vi "Determine Sector Edge Location.vi"(11 "Preanalysis Stage":bool) -> (2 "Left Sector Edge":u8, 3 "Right Sector Edge":u8)   [LabVIEW 2013]
doc: "Takes the average sector intensities and compares each average to the threshold value to determine which sector the edge is located in."
uses:
  Globals/Accumulated Sector Intensity.vi
  Globals/Sector Parameter Global.vi
  <vilib>/rvi/FIFO/Fifo_Resource/nirvififoEmulationReadFpgaImpl.vi
  <vilib>/rvi/DataTransferAndStorage/Container/Common/niFpgaContainerGetUniqueNameForEmu.vi
  <vilib>/rvi/interface/RandomDataEmulation/nirviRandomDataFPGAFIFO.vi
  <vilib>/rvi/interface/RandomDataEmulation/niFpgaRandomDataHandleErrors.vi
  <vilib>/rvi/DataTransferAndStorage/Container/XNode/niFpgaContainer.xnode
  <vilib>/rvi/FIFO/Fifo_Resource/nirvififoEmulationRead.vi
  <vilib>/rvi/interface/RandomDataEmulation/nirviRandomDataFpgaReadWriteTemplate.vi
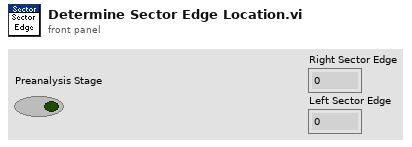
[diagram p1: front panel]
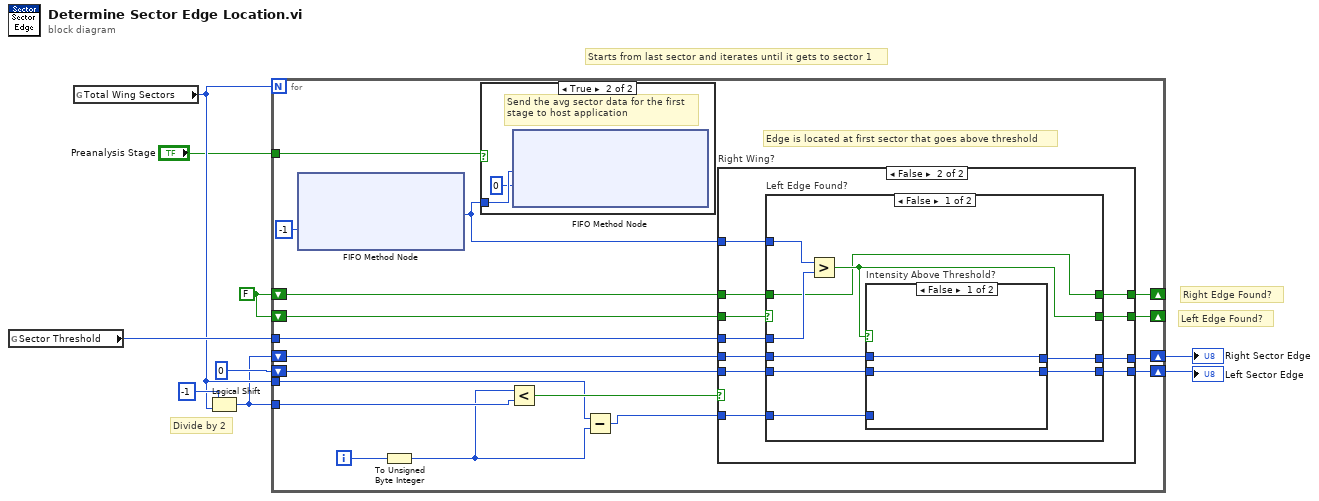
[diagram p0: block diagram]
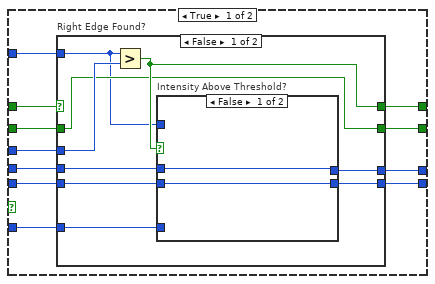
[diagram p3: hidden frame]
diagram:
  w6 = FALSE ("Left Edge Found?")
  # "Starts from last sector and iterates until it gets to sector 1"
  # "Left Edge Found?"
  # "Right Edge Found?"
  # "Divide by 2"
  n1 = global read "Sector Parameter Global.vi" "Sector Threshold"() -> (w4:u8)
  n2 = global read "Accumulated Sector Intensity.vi" "Total Wing Sectors"() -> (w3:u8)
  n3 = Logical Shift(y=i16 -1, x=w3) -> (x << y=w1:u8)
  n4 = for {
    N: w3 -> [_]
    tunnel: w4 -> [w25]
    tunnel: w1 -> [w26]
    shift-right: [w23] -> _
    shift-left: w6 -> [w24]
    shift-right: [w16] -> _
    shift-left: w6 -> [w17]
    shift-right: [w21] -> w9
    shift-left: w1 -> [w20]
    shift-right: [w19] -> w8
    shift-left: u8 0 ("Total Wing Sectors") -> [w18]
    tunnel: w3 -> [w13]
    tunnel: "Preanalysis Stage" -> [w10]
    i -> [w22]
    # "Edge is located at first sector that goes above threshold"
    n5 = xnode ("FIFO Method Node")("Timeout"=-1) -> ("Element"=w15:u8)  [unwired: 1 in, 2 out]
    n6 = To Unsigned Byte Integer(number=w22) -> (unsigned 8bit integer=w12:u8)
    n7 = case shown="True" w10 {
      tunnel: w15 -> [_ w29]
      frame False {
      }
      frame True {
        # "Send the avg sector data for the first\nstage to host application"
        n8 = xnode ("FIFO Method Node")("Element"=w29, "Timeout"=0) -> ()  [unwired: 1 in, 2 out]
      }
    }
    n9 = Less?(x=w12, y=w26) -> (x < y?=w27:bool)
    n10 = Subtract(x=w13, y=w12) -> (x-y=w11:u8)
    n11 = case "Right Wing?" shown="False" w27 {
      tunnel: w15 -> [w39 w68]
      tunnel: w25 -> [w38 w67]
      tunnel: w24 -> [w40 w59]
      tunnel: [w37 w66] -> w23
      tunnel: w11 -> [w36 w65]
      tunnel: [w35 w64] -> w21
      tunnel: w20 -> [w34 w63]
      tunnel: [w33 w62] -> w19
      tunnel: w18 -> [w32 w61]
      tunnel: w17 -> [w31 w60]
      tunnel: [w30 w58] -> w16
      frame True {
        n12 = case "Right Edge Found?" shown="False" w40 {
          selector: w40 -> [_ w54]
          tunnel: w39 -> [w41 _]
          tunnel: w38 -> [w49 _]
          tunnel: [w48 w54] -> w37
          tunnel: w36 -> [w47 _]
          tunnel: [w46 w57] -> w35
          tunnel: w34 -> [w45 w57]
          tunnel: [w44 w56] -> w33
          tunnel: w32 -> [w43 w56]
          tunnel: w31 -> [w42 w55]
          tunnel: [w42 w55] -> w30
          frame False {
            n13 = Greater?(x=w41, y=w49) -> (0:w48:bool)
            n14 = case "Intensity Above Threshold?" shown="False" w48 {
              tunnel: w47 -> [_ w52]
              tunnel: [w51 w52] -> w46
              tunnel: w45 -> [w51 _]
              tunnel: [w50 w53] -> w44
              tunnel: w43 -> [w50 w53]
              tunnel: w41 -> [_ _]
              frame False {
              }
              frame True {
              }
            }
          }
          frame True {
          }
        }
      }
      frame False {
        n15 = case "Left Edge Found?" shown="False" w60 {
          selector: w60 -> [_ w82]
          tunnel: w68 -> [w69 _]
          tunnel: w67 -> [w77 _]
          tunnel: [w70 w83] -> w66
          tunnel: w65 -> [w76 _]
          tunnel: [w75 w85] -> w64
          tunnel: w63 -> [w74 w85]
          tunnel: [w73 w84] -> w62
          tunnel: w61 -> [w72 w84]
          tunnel: w59 -> [w70 w83]
          tunnel: [w71 w82] -> w58
          frame False {
            n16 = Greater?(x=w69, y=w77) -> (0:w71:bool)
            n17 = case "Intensity Above Threshold?" shown="False" w71 {
              tunnel: w76 -> [_ w80]
              tunnel: [w79 w81] -> w75
              tunnel: w74 -> [w79 w81]
              tunnel: [w78 w80] -> w73
              tunnel: w72 -> [w78 _]
              frame False {
              }
              frame True {
              }
            }
          }
          frame True {
          }
        }
      }
    }
  }
  "Right Sector Edge" <- w9
  "Left Sector Edge" <- w8
